vi "setConfigArray.vi"(8 "error in (no error)":errorcluster, 10 "ConfigArray":T1(array[cluster]), 11 "EthernetSupply in":refnum<class "EthernetSupply.lvclass">) -> (0 "error out":errorcluster, 3 "EthernetSupply out":refnum<class "EthernetSupply.lvclass">)   [LabVIEW 2009, in "Tools.lvlib" / "DatabaseHelpers.lvlib" / "EthernetSupply.lvclass"]
uses:
  EthernetSupply.lvclass
  EthernetSupply.lvclass/EthernetSupply.ctl
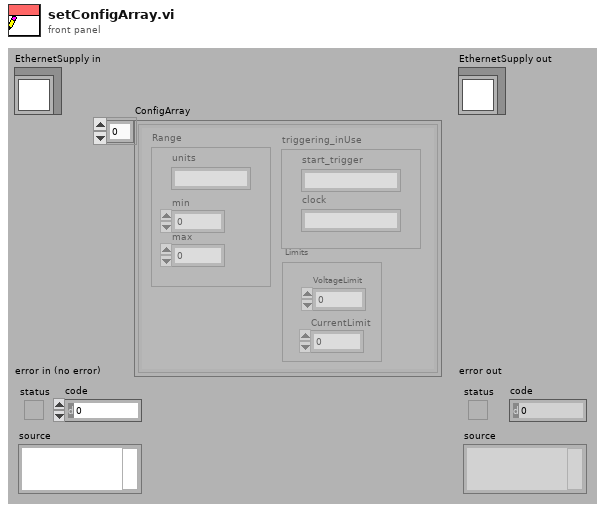
[diagram p1: front panel]
types:
  T1 = cluster{"Range":cluster{"units":string, "min":dbl, "max":dbl}, "triggering_inUse":cluster{"start_trigger":string, "clock":string}, "Limits":cluster{"VoltageLimit":dbl, "CurrentLimit":dbl}}[]
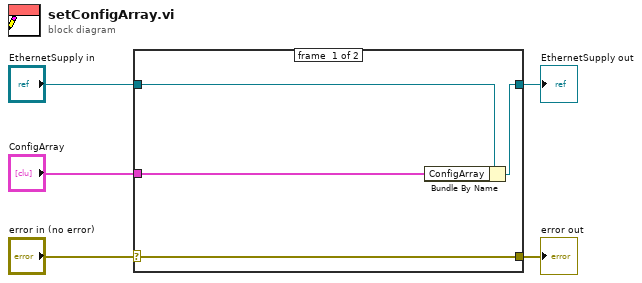
[diagram p0: block diagram]
diagram:
  n1 = case shown="No Error" "error in (no error)" {
    selector: "error in (no error)" -> [w9 w10]
    tunnel: [w9 w10] -> w4
    tunnel: [w7 w11] -> w2
    tunnel: "EthernetSupply in" -> [w8 w11]
    tunnel: "ConfigArray" -> [w6 _]
    frame #0 {
      n2 = Bundle By Name(cluster=w8, "ConfigArray"=w6) -> (w7:refnum<class "EthernetSupply.lvclass">)
    }
    frame #1 {
    }
  }
  "error out" <- w4
  "EthernetSupply out" <- w2
